vi "TCP-IP-Dialog.vi"() -> (2 "serial number":string, 3 "IP address+ port":string, 4 "cancelled":bool)   [LabVIEW 2013]
panel:
  in  "rescan":bool
  in  "available devices":i32(listbox)
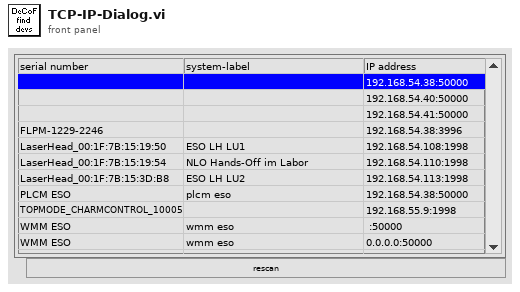
[diagram p1: front panel]
types:
  T1 = cluster{"serial-number":string, "firmware-version":string, "DeCoF-version":string, "system-type":string, "system-model":string, "system-label":string, "system-features":i32, "ip-addr":string, "cmd-port":i32, "monitor-port":i32}[]
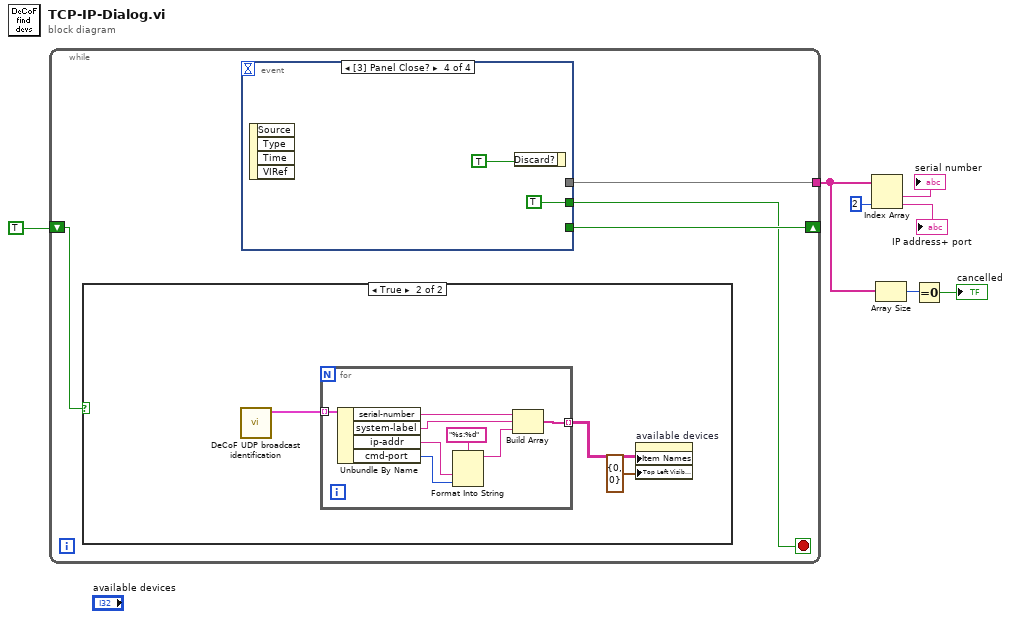
[diagram p0: block diagram]
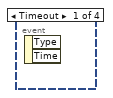
[diagram p2: hidden frame]
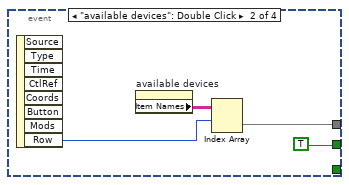
[diagram p3: hidden frame]
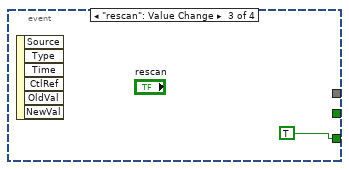
[diagram p4: hidden frame]
diagram:
  n1 = while {
    shift-right: [w10] -> _
    shift-left: TRUE -> [w11]
    tunnel: [w8] -> w3
    stop <- w9 stop-if-true
    n2 = case shown="True" w11 {
      frame False {
      }
      frame True {
        n3 = call "DeCoF UDP broadcast identification.vi"() -> ("device list"=w20:T1)  [unwired: 5 in, 4 out]
        n4 = for {
          tunnel: w20 -> [w29] mode=indexing
          tunnel: [w26] -> w19 mode=indexing
          n5 = Unbundle By Name(w29) -> ("serial-number"=w28:string, "system-label"=w27:string, "ip-addr"=w24:string, "cmd-port"=w23:i32)
          n6 = Format Into String(format string="%s:%d", w24, w23) -> (resulting string=w22:string)  [unwired: 2 in, 1 out]
          n7 = Build Array(w28, w27, w22) -> (w26:string[])
        }
        n8 = property on="available devices" class="MCListbox (strict)"("Item Names"=w19, "Top Left Visible Cell"=cluster{"Row":i32, "Column":i32} {"Row"=0, "Column"=0} ("Active Cell")) -> ()  [unwired: 2 in, 2 out]
      }
    }
    n9 = event shown="[3] Panel Close?" {
      selector: _ -> [_ _ _ _]
      dyn-events: _ -> [_ _ _ _]
      timeout: _ -> [_ _ _ _]
      tunnel: [_ _ TRUE _] -> w10
      tunnel: [_ TRUE _ TRUE] -> w9
      tunnel: [_ w13 _ _] -> w8
      event Timeout {
        n10 = event-data() -> ()  [unwired: 1 in, 2 out]
      }
      event "available devices": Double Click {
        n11 = event-data() -> ("Row"=w14:i32)  [unwired: 1 in, 7 out]
        n12 = property on="available devices" class="MCListbox (strict)"() -> ("Item Names"=w15:string[][])  [unwired: 2 in, 2 out]
        n13 = Index Array(array=w15, index (row)=w14) -> (element=w13:string[])  [unwired: 1 in]
      }
      event "rescan": Value Change {
        n14 = event-data() -> ()  [unwired: 1 in, 6 out]
      }
      event Panel Close? {
        n15 = event-data() -> ()  [unwired: 1 in, 4 out]
        n16 = event-data("Discard?"=TRUE) -> ()  [unwired: 1 in, 1 out]
      }
    }
  }
  n17 = Index Array(array=w3, index #2=2 ("index")) -> (element #1=→"serial number":string, element #2=→"IP address+ port":string)  [unwired: 1 in]
  n18 = Array Size(array=w3) -> (size(s)=w2:i32)
  n19 = Equal To 0?(x=w2) -> (x = 0?=→"cancelled":bool)
